vi "KMCS2000 380-780 array.vi"() -> (3 "Array":i32[](array[numeric]))   [LabVIEW 2018]
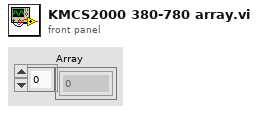
[diagram p1: front panel]
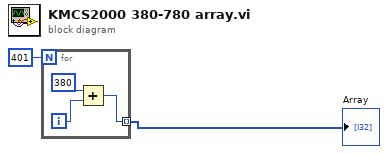
[diagram p0: block diagram]
diagram:
  n1 = for {
    N: 401 -> [_]
    tunnel: [w3] -> w2 mode=indexing
    i -> [w5]
    n2 = Add(x=380, y=w5) -> (x+y=w3:i32)
  }
  "Array" <- w2
